vi "Collector.vi"(0 "CollectorAction":T1, 1 "Raise":dbl, 5 "CollectorMotor":string="My Motor RefNum", 7 "TopLS":string="My DigitalInput RefNum", 9 "BottomLS":string="My DigitalInput RefNum", 11 "Error in":errorcluster, 12 "Lower":dbl) -> (6 "Upper Triggered?":bool, 10 "Lower Triggered?":bool, 15 "Error out":errorcluster)   [LabVIEW 2013]
doc: "Will Raise, Lower, or Stop the collector motor if a button is pressed for either, and will stop if hit by a limit switch."
uses:
  CollectorEnum.ctl
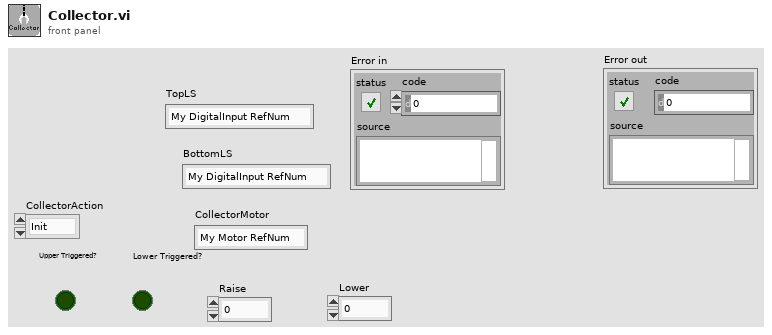
[diagram p1: front panel]
types:
  T1 = typedef "CollectorEnum.ctl" = enum16{"Init", "Raise", "Lower", "Stop", "GetStatus"}
  T2 = typedef "WPI_MotorControlDeviceRef.ctl" = cluster{"DeviceStatus":errorcluster, "Type":enum16{"PWM", "CAN"}, "PWM":cluster{"Digital Module":T3, "PWM Channel":T4, "DeadBand":T5}, "CAN":cluster{"Device Number":u8, "Control Mode":T6, "Semaphore":T7, "Max Vout":dbl}, "Invert":bool, "TransformRef":T8, "InvTransformRef":T8}
  T3 = typedef "FPGA_TypedefDigitalModule.ctl" = enum16{"Digital Module 1", "Digital Module 2"}
  T4 = typedef "FPGA_DIOPWMChannel.ctl" = enum8{"PWM 1", "PWM 2", "PWM 3", "PWM 4", "PWM 5", "PWM 6", "PWM 7", "PWM 8", "PWM 9", "PWM 10", "Invalid"}
  T5 = typedef "WPI_PWMDeadband.ctl" = cluster{"Name":string, "maxPositivePwm":i32, "minPositivePwm":i32, "centerPwm":i32, "maxNegativePwm":i32, "minNegativePwm":i32, "angularRange":u16}
  T6 = typedef "WPI_CANJaguar_ControlMode.ctl" = enum8{"Percent VBus", "Current", "Speed", "Position", "Voltage"}
  T7 = typedef "Semaphore RefNum" = refnum<k1>
  T8 = typedef "WPI_PWMTransform_ConPane.ctl" = refnum<vi>
  T9 = typedef "WPI_DigitalInputDevRef.ctl" = cluster{"DevStatus":errorcluster, "DIO Channel":T10, "Digital Module":T3}
  T10 = typedef "FPGA_DIOChannel.ctl" = enum8{"DIO 1", "DIO 2", "DIO 3", "DIO 4", "DIO 5", "DIO 6", "DIO 7", "DIO 8", "DIO 9", "DIO 10", "DIO 11", "DIO 12", "DIO 13", "DIO 14", "Invalid"}
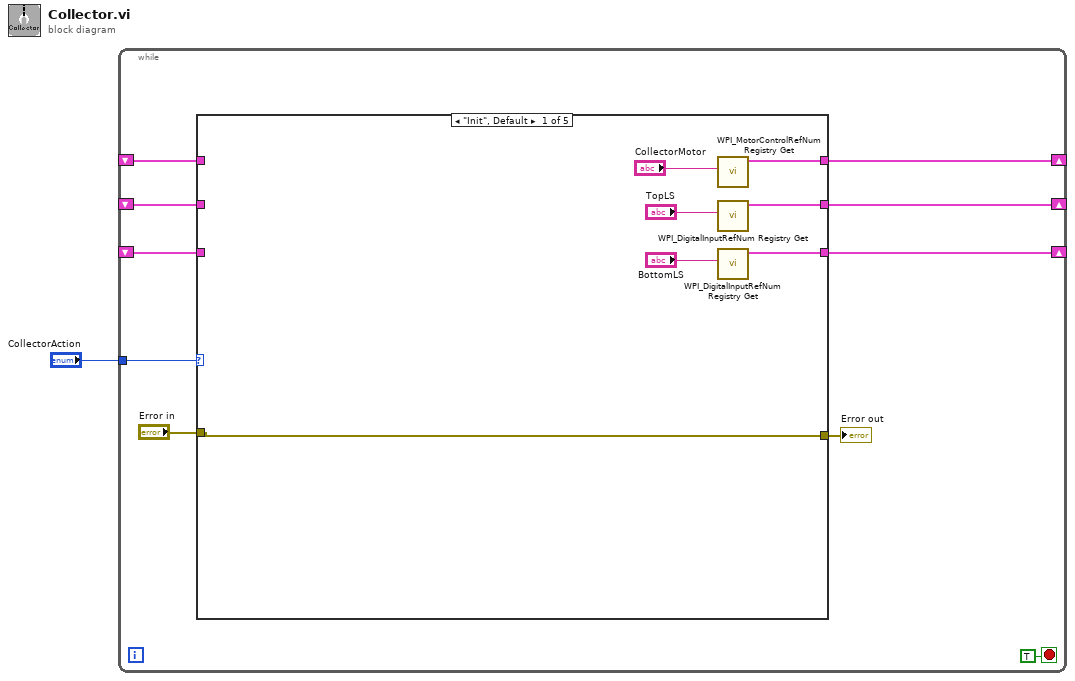
[diagram p0: block diagram]
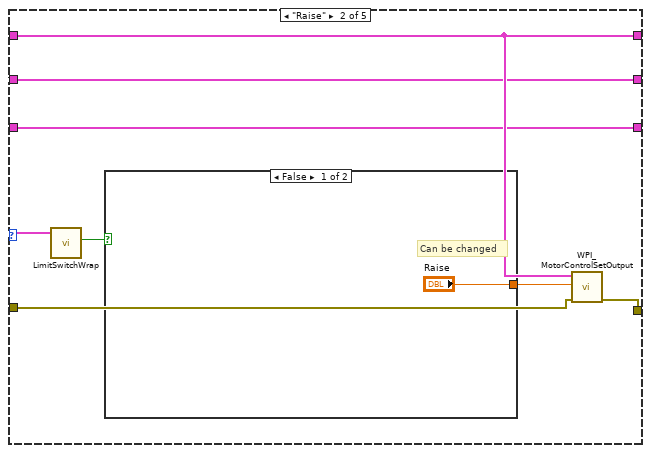
[diagram p2: hidden frame]
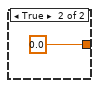
[diagram p3: hidden frame]
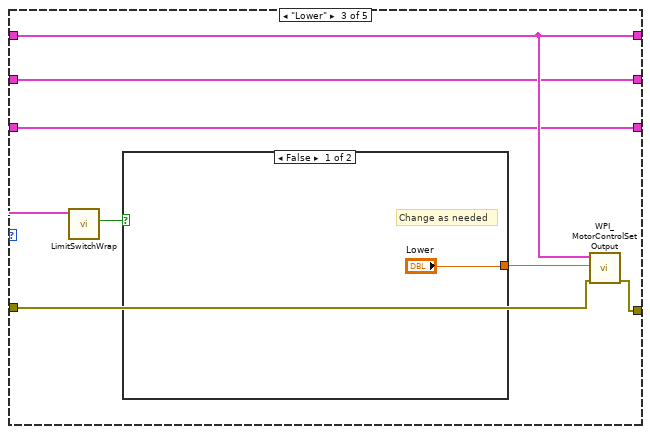
[diagram p4: hidden frame]
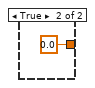
[diagram p5: hidden frame]
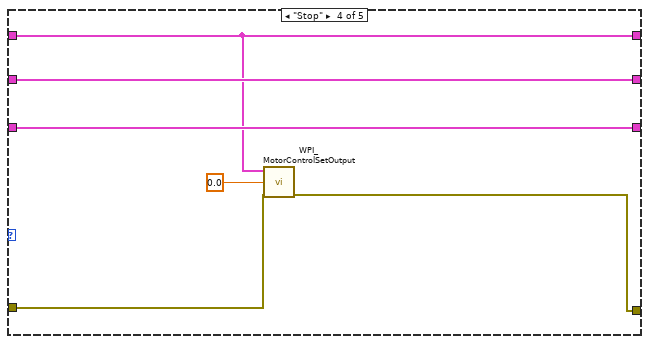
[diagram p6: hidden frame]
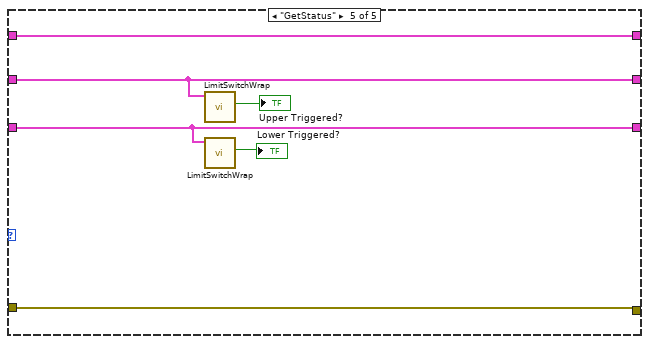
[diagram p7: hidden frame]
diagram:
  n1 = while {
    tunnel: "CollectorAction" -> [w11]
    shift-right: [w7] -> _
    shift-left: _ -> [w4]
    shift-right: [w8] -> _
    shift-left: _ -> [w5]
    shift-right: [w9] -> _
    shift-left: _ -> [w6]
    stop <- TRUE stop-if-true
    n2 = case shown="\"Init\", Default" w11 {
      tunnel: [w18 w23 w32 w39 w48] -> w9
      tunnel: [w17 w21 w31 w41 w47] -> w8
      tunnel: [w16 w22 w30 w40 w46] -> w7
      tunnel: w6 -> [_ w23 w32 w39 w48]
      tunnel: w5 -> [_ w21 w31 w41 w47]
      tunnel: w4 -> [_ w22 w30 w40 w46]
      tunnel: "Error in" -> [w12 w20 w29 w38 w43]
      tunnel: [w12 w19 w28 w37 w43] -> w2
      frame "Init", Default {
        n3 = call <vilib>:"WPI_MotorControlRefNum Registry Get.vi"("refnum name"="CollectorMotor") -> ("MotorControlDevRef"=w18:T2)  [unwired: 9 in, 1 out]
        n4 = call <vilib>:"WPI_DigitalInputRefNum Registry Get.vi"("refnum name"="TopLS") -> ("DigitalInputDevRef"=w17:T9)  [unwired: 9 in, 1 out]
        n5 = call <vilib>:"WPI_DigitalInputRefNum Registry Get.vi"("refnum name"="BottomLS") -> ("DigitalInputDevRef"=w16:T9)  [unwired: 9 in, 1 out]
      }
      frame "Raise" {
        n6 = call "LimitSwitchWrap.vi"("DigitalInputDevRef"=w21) -> ("Triggered"=w25:bool)  [unwired: 9 in, 1 out]
        n7 = case shown="False" w25 {
          tunnel: ["Raise" 0.0] -> w24
          frame False {
            # "Can be changed"
          }
          frame True {
          }
        }
        n8 = call <vilib>:"WPI_MotorControlSetOutput.vi"("error in (no error)"=w20, "Output"=w24, "MotorControlDevRef"=w23) -> ("error out"=w19:errorcluster)  [unwired: 6 in, 2 out]
      }
      frame "Lower" {
        n9 = call "LimitSwitchWrap.vi"("DigitalInputDevRef"=w30) -> ("Triggered"=w34:bool)  [unwired: 9 in, 1 out]
        n10 = case shown="False" w34 {
          tunnel: ["Lower" 0.0] -> w33
          frame False {
            # "Change as needed"
          }
          frame True {
          }
        }
        n11 = call <vilib>:"WPI_MotorControlSetOutput.vi"("error in (no error)"=w29, "Output"=w33, "MotorControlDevRef"=w32) -> ("error out"=w28:errorcluster)  [unwired: 6 in, 2 out]
      }
      frame "Stop" {
        n12 = call <vilib>:"WPI_MotorControlSetOutput.vi"("error in (no error)"=w38, "Output"=0.0, "MotorControlDevRef"=w39) -> ("error out"=w37:errorcluster)  [unwired: 6 in, 2 out]
      }
      frame "GetStatus" {
        n13 = call "LimitSwitchWrap.vi"("DigitalInputDevRef"=w47) -> ("Triggered"=→"Upper Triggered?":bool)  [unwired: 9 in, 1 out]
        n14 = call "LimitSwitchWrap.vi"("DigitalInputDevRef"=w46) -> ("Triggered"=→"Lower Triggered?":bool)  [unwired: 9 in, 1 out]
      }
    }
    "Error out" <- w2
  }
